vi "Teleop.vi"(10 "Match Info":T1={"Autonomous Elapsed Seconds"=0.0, "TeleOp Elapsed Seconds"=0.0, "Disabled Elapsed Seconds"=0.0, "Visited Autonomous"=FALSE, "Visited TeleOp"=FALSE, "Visited Disabled"=FALSE, "Autonomous Settings"={"Autonomous Style"=enum."Independent", "VI Refnum"=refnum}}, 11 "Call Context":T2) -> ()   [LabVIEW 2012]
doc: "This VI is called for each TeleOp packet received from the DS where the robot is not disabled. It is often used to read from the joysticks and update I/O or to update setpoints for timed control loops. It should complete and return within 20 milliseconds or it may miss DS packets."
uses:
  <vilib>/Rock Robotics/WPI/DriverStation/WPI_DriverStationDerivedRobotMode.ctl
  <vilib>/Rock Robotics/WPI/DriverStation/WPI_DriverStationMatch Info.ctl
  Robot Global Data.vi
  <vilib>/addons/control/pid/pid.llb/PID (DBL).vi
  <vilib>/Rock Robotics/WPI/Joystick/WPI_JoystickGetSetRefNum.vi
  <vilib>/addons/control/pid/NI_PID_pid.lvlib
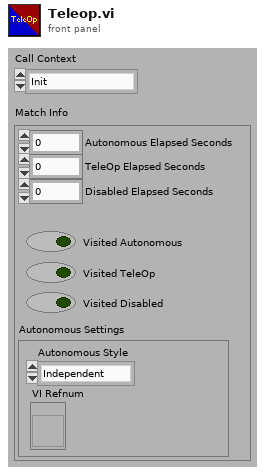
[diagram p1: front panel]
types:
  T1 = typedef "WPI_DriverStationMatch Info.ctl" = cluster{"Autonomous Elapsed Seconds":dbl, "TeleOp Elapsed Seconds":dbl, "Disabled Elapsed Seconds":dbl, "Visited Autonomous":bool, "Visited TeleOp":bool, "Visited Disabled":bool, "Autonomous Settings":cluster{"Autonomous Style":enum16{"Iterative", "Independent"}, "VI Refnum":refnum<vi>}}
  T2 = typedef "WPI_DriverStationDerivedRobotMode.ctl" = enum16{"Init", "Execute", "Stop"}
  T3 = cluster{"proportional gain (Kc)":dbl, "integral time (Ti, min)":dbl, "derivative time (Td, min)":dbl}
  T4 = typedef "WPI_JoystickDevRef.ctl" = cluster{"Device":T5}
  T5 = typedef "WPI_JoystickDeviceEnum.ctl" = enum16{"USB 1", "USB 2", "USB 3", "USB 4", "Kinect 1", "Kinect 2"}
  T6 = typedef "WPI_JoystickButtonState.ctl" = cluster{"Button 1":bool, "Button 2":bool, "Button 3":bool, "Button 4":bool, "Button 5":bool, "Button 6":bool, "Button 7":bool, "Button 8":bool, "Button 9":bool, "Button 10":bool, "Button 11":bool, "Button 12":bool}
  T7 = cluster{"axis 1 (x)":dbl, "axis 2 (y)":dbl, "axis 3 (throttle)":dbl, "axis 4":dbl, "axis 5":dbl, "axis 6":dbl}
  T8 = typedef "WPI_MotorControlDeviceRef.ctl" = cluster{"DeviceStatus":errorcluster, "Type":enum16{"PWM", "CAN"}, "PWM":cluster{"Digital Module":T9, "PWM Channel":T10, "DeadBand":T11}, "CAN":cluster{"Device Number":u8, "Control Mode":T12, "Semaphore":T13, "Max Vout":dbl}, "Invert":bool, "TransformRef":T14, "InvTransformRef":T14}
  T9 = typedef "FPGA_TypedefDigitalModule.ctl" = enum16{"Digital Module 1", "Digital Module 2"}
  T10 = typedef "FPGA_DIOPWMChannel.ctl" = enum8{"PWM 1", "PWM 2", "PWM 3", "PWM 4", "PWM 5", "PWM 6", "PWM 7", "PWM 8", "PWM 9", "PWM 10", "Invalid"}
  T11 = typedef "WPI_PWMDeadband.ctl" = cluster{"Name":string, "maxPositivePwm":i32, "minPositivePwm":i32, "centerPwm":i32, "maxNegativePwm":i32, "minNegativePwm":i32, "angularRange":u16}
  T12 = typedef "WPI_CANJaguar_ControlMode.ctl" = enum8{"Percent VBus", "Current", "Speed", "Position", "Voltage"}
  T13 = typedef "Semaphore RefNum" = refnum<k1>
  T14 = typedef "WPI_PWMTransform_ConPane.ctl" = refnum<vi>
  T15 = typedef "WPI_AnalogChannelDevRef.ctl" = cluster{"DevStatus":errorcluster, "Analog Module":T16, "Analog Channel":T17}
  T16 = typedef "FPGA_TypedefAnalogModule.ctl" = enum16{"Analog Module 1", "Analog Module 2"}
  T17 = typedef "FPGA_AIChannel.ctl" = enum8{"AI 1", "AI 2", "AI 3", "AI 4", "AI 5", "AI 6", "AI 7", "AI 8", "Invalid"}
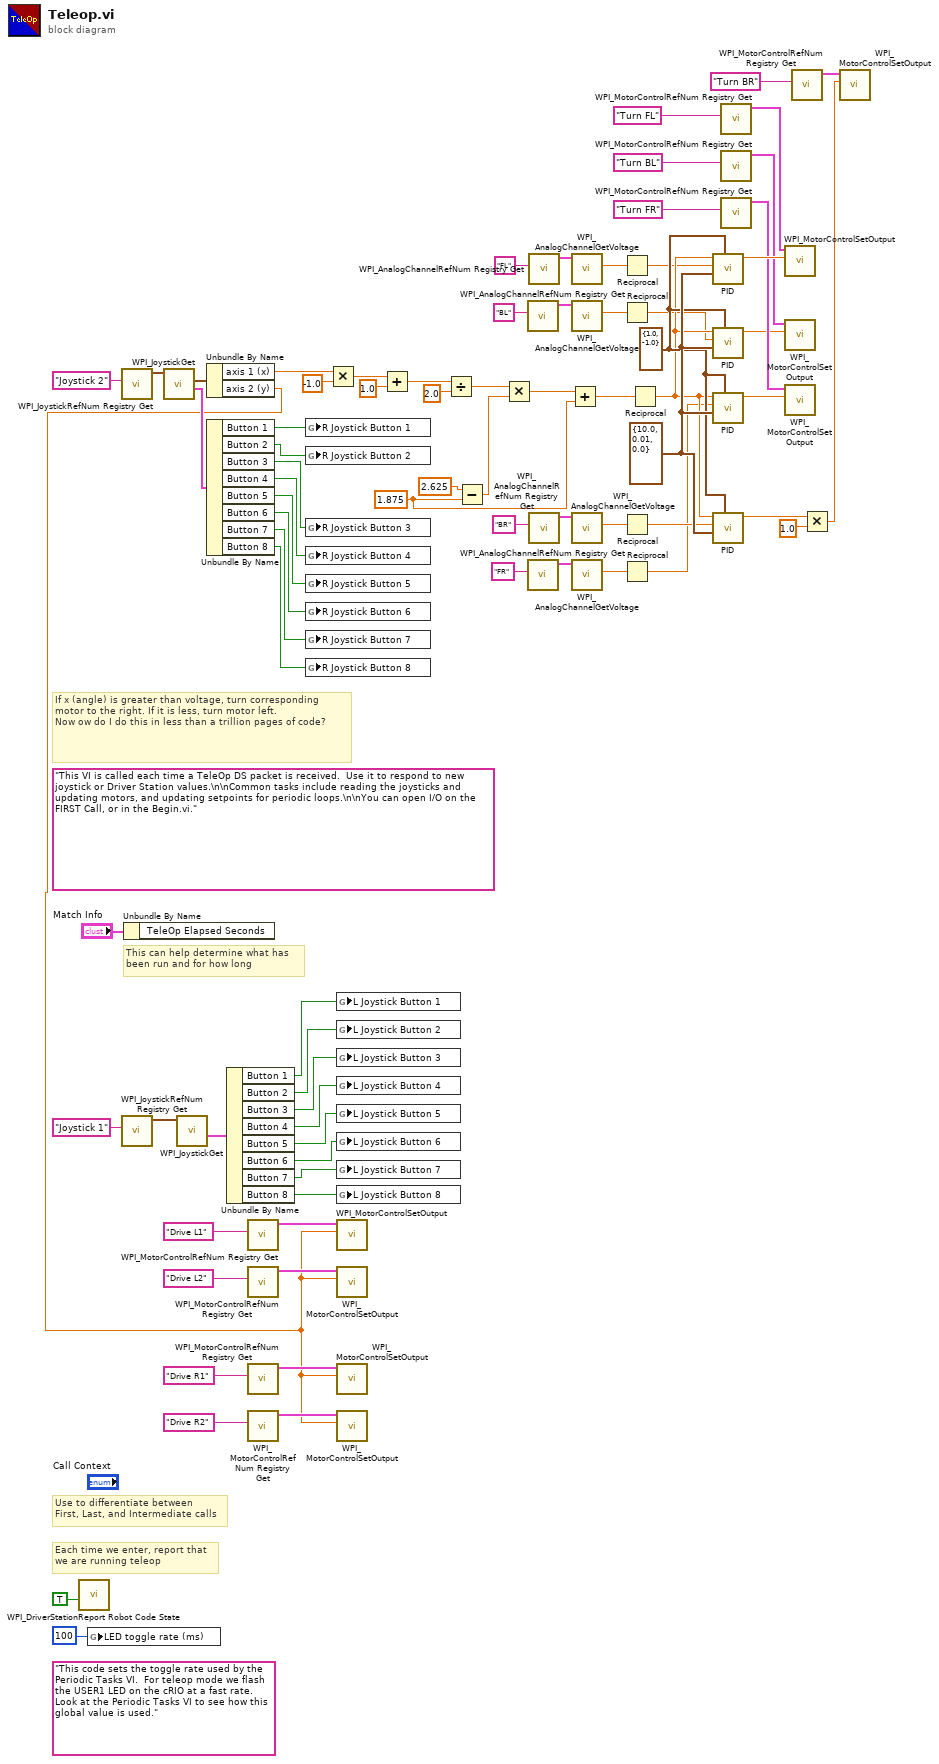
[diagram p0: block diagram]
diagram:
  w21 = T3 {"proportional gain (Kc)"=10.0, "integral time (Ti, min)"=0.01, "derivative time (Td, min)"=0.0} ("PID gains")
  w20 = cluster{"output high":dbl, "output low":dbl} {"output high"=1.0, "output low"=-1.0} ("output range")
  w19 = 1.875 ("y")
  (unwired) "This code sets the toggle rate used by the Periodic Tasks VI.  For teleop mode we flash the USER1 LED on the cRIO at a fast rate.  Look at the Periodic Tasks VI to see how this global value is used."
  (unwired) "This VI is called each time a TeleOp DS packet is received.  Use it to respond to new joystick or Driver Station values.\n\nCommon tasks include reading the joysticks and updating motors, and updating setpoints for periodic loops.\n\nYou can open I/O on the FIRST Call, or in the Begin.vi."
  # "If x (angle) is greater than voltage, turn corresponding motor to the right. If it is less, turn motor left.\nNow ow do I do this in less than a trillion pages of code?"
  # "Each time we enter, report that\nwe are running teleop"
  # "Use to differentiate between\nFirst, Last, and Intermediate calls"
  # "This can help determine what has\nbeen run and for how long"
  n1 = call <vilib>:"WPI_DriverStationReport Robot Code State.vi"("TeleOp"=TRUE ("Autonomous")) -> ()  [unwired: 10 in, 1 out]
  n2 = global write "Robot Global Data.vi" "LED toggle rate (ms)"(u32 100 ("LED ms toggle rate")) -> ()
  n3 = call <vilib>:"WPI_JoystickRefNum Registry Get.vi"("refnum name"="Joystick 2") -> ("JoystickDevRef"=w73:T4)  [unwired: 1 in, 9 out]
  n4 = call <vilib>:"WPI_JoystickRefNum Registry Get.vi"("refnum name"="Joystick 1") -> ("JoystickDevRef"=w78:T4)  [unwired: 1 in, 9 out]
  n5 = Unbundle By Name("Match Info") -> ()  [unwired: 1 out]
  n6 = call <vilib>:"WPI_JoystickGet.vi"("JoystickDevRef"=w73) -> ("Buttons"=w72:T6, "Axes"=w75:T7)  [unwired: 1 in, 4 out]
  n7 = call <vilib>:"WPI_JoystickGet.vi"("JoystickDevRef"=w78) -> ("Buttons"=w71:T6)  [unwired: 1 in, 5 out]
  n8 = Unbundle By Name(w75) -> ("axis 1 (x)"=w11:dbl, "axis 2 (y)"=w1:dbl)
  n9 = Unbundle By Name(w72) -> ("Button 1"=w62:bool, "Button 2"=w61:bool, "Button 3"=w60:bool, "Button 4"=w59:bool, "Button 5"=w58:bool, "Button 6"=w57:bool, "Button 7"=w56:bool, "Button 8"=w55:bool)
  n10 = Unbundle By Name(w71) -> ("Button 1"=w70:bool, "Button 2"=w69:bool, "Button 3"=w68:bool, "Button 4"=w67:bool, "Button 5"=w66:bool, "Button 6"=w65:bool, "Button 7"=w64:bool, "Button 8"=w63:bool)
  n11 = call <vilib>:"WPI_MotorControlRefNum Registry Get.vi"("refnum name"="Drive L1") -> ("MotorControlDevRef"=w47:T8)  [unwired: 9 in, 1 out]
  n12 = call <vilib>:"WPI_MotorControlRefNum Registry Get.vi"("refnum name"="Drive L2") -> ("MotorControlDevRef"=w46:T8)  [unwired: 9 in, 1 out]
  n13 = call <vilib>:"WPI_MotorControlRefNum Registry Get.vi"("refnum name"="Drive R1") -> ("MotorControlDevRef"=w45:T8)  [unwired: 9 in, 1 out]
  n14 = call <vilib>:"WPI_MotorControlRefNum Registry Get.vi"("refnum name"="Drive R2") -> ("MotorControlDevRef"=w44:T8)  [unwired: 9 in, 1 out]
  n15 = global write "Robot Global Data.vi" "R Joystick Button 1"(w62) -> ()
  n16 = global write "Robot Global Data.vi" "R Joystick Button 2"(w61) -> ()
  n17 = global write "Robot Global Data.vi" "R Joystick Button 3"(w60) -> ()
  n18 = global write "Robot Global Data.vi" "R Joystick Button 4"(w59) -> ()
  n19 = global write "Robot Global Data.vi" "R Joystick Button 5"(w58) -> ()
  n20 = global write "Robot Global Data.vi" "R Joystick Button 6"(w57) -> ()
  n21 = global write "Robot Global Data.vi" "R Joystick Button 7"(w56) -> ()
  n22 = global write "Robot Global Data.vi" "R Joystick Button 8"(w55) -> ()
  n23 = Multiply(x=w11, y=-1.0) -> (x*y=w10:dbl)
  n24 = global write "Robot Global Data.vi" "L Joystick Button 1"(w70) -> ()
  n25 = global write "Robot Global Data.vi" "L Joystick Button 2"(w69) -> ()
  n26 = global write "Robot Global Data.vi" "L Joystick Button 3"(w68) -> ()
  n27 = global write "Robot Global Data.vi" "L Joystick Button 4"(w67) -> ()
  n28 = global write "Robot Global Data.vi" "L Joystick Button 5"(w66) -> ()
  n29 = global write "Robot Global Data.vi" "L Joystick Button 6"(w65) -> ()
  n30 = global write "Robot Global Data.vi" "L Joystick Button 7"(w64) -> ()
  n31 = global write "Robot Global Data.vi" "L Joystick Button 8"(w63) -> ()
  n32 = call <vilib>:"WPI_MotorControlSetOutput.vi"("Output"=w1, "MotorControlDevRef"=w47) -> ()  [unwired: 7 in, 3 out]
  n33 = call <vilib>:"WPI_MotorControlSetOutput.vi"("Output"=w1, "MotorControlDevRef"=w46) -> ()  [unwired: 7 in, 3 out]
  n34 = call <vilib>:"WPI_MotorControlSetOutput.vi"("Output"=w1, "MotorControlDevRef"=w45) -> ()  [unwired: 7 in, 3 out]
  n35 = call <vilib>:"WPI_MotorControlSetOutput.vi"("Output"=w1, "MotorControlDevRef"=w44) -> ()  [unwired: 7 in, 3 out]
  n36 = Add(x=w10, y=1.0) -> (x+y=w42:dbl)
  n37 = Divide(x=w42, y=2.0) -> (x/y=w38:dbl)
  n38 = Subtract(x=2.625, y=w19) -> (x-y=w39:dbl)
  n39 = Multiply(x=w38, y=w39) -> (x*y=w40:dbl)
  n40 = call <vilib>:"WPI_AnalogChannelRefNum Registry Get.vi"("refnum name"="BL") -> ("AIDeviceRef"=w26:T15)  [unwired: 9 in, 1 out]
  n41 = call <vilib>:"WPI_AnalogChannelRefNum Registry Get.vi"("refnum name"="FR") -> ("AIDeviceRef"=w31:T15)  [unwired: 9 in, 1 out]
  n42 = call <vilib>:"WPI_AnalogChannelRefNum Registry Get.vi"("refnum name"="FL") -> ("AIDeviceRef"=w36:T15)  [unwired: 9 in, 1 out]
  n43 = call <vilib>:"WPI_AnalogChannelRefNum Registry Get.vi"("refnum name"="BR") -> ("AIDeviceRef"=w54:T15)  [unwired: 9 in, 1 out]
  n44 = Add(x=w40, y=w19) -> (x+y=w9:dbl)
  n45 = call <vilib>:"WPI_AnalogChannelGetVoltage.vi"("AIDeviceRef"=w36) -> ("Voltage"=w3:dbl)  [unwired: 8 in, 2 out]
  n46 = call <vilib>:"WPI_AnalogChannelGetVoltage.vi"("AIDeviceRef"=w26) -> ("Voltage"=w7:dbl)  [unwired: 8 in, 2 out]
  n47 = call <vilib>:"WPI_AnalogChannelGetVoltage.vi"("AIDeviceRef"=w54) -> ("Voltage"=w14:dbl)  [unwired: 8 in, 2 out]
  n48 = call <vilib>:"WPI_AnalogChannelGetVoltage.vi"("AIDeviceRef"=w31) -> ("Voltage"=w5:dbl)  [unwired: 8 in, 2 out]
  n49 = Reciprocal(x=w3) -> (1/x=w2:dbl)
  n50 = Reciprocal(x=w7) -> (1/x=w6:dbl)
  n51 = Reciprocal(x=w14) -> (1/x=w13:dbl)
  n52 = Reciprocal(x=w5) -> (1/x=w4:dbl)
  n53 = Reciprocal(x=w9) -> (1/x=w8:dbl)
  n54 = call-poly <vilib>:"PID.vi"("output range"=w20, "PID gains"=w21, "process variable"=w2, "setpoint"=w8) -> ("output"=w33:dbl)  [unwired: 6 in, 1 out]
  n55 = call-poly <vilib>:"PID.vi"("output range"=w20, "PID gains"=w21, "process variable"=w6, "setpoint"=w8) -> ("output"=w23:dbl)  [unwired: 6 in, 1 out]
  n56 = call-poly <vilib>:"PID.vi"("output range"=w20, "PID gains"=w21, "process variable"=w4, "setpoint"=w8) -> ("output"=w28:dbl)  [unwired: 6 in, 1 out]
  n57 = call-poly <vilib>:"PID.vi"("output range"=w20, "PID gains"=w21, "process variable"=w13, "setpoint"=w8) -> ("output"=w16:dbl)  [unwired: 6 in, 1 out]
  n58 = call <vilib>:"WPI_MotorControlRefNum Registry Get.vi"("refnum name"="Turn FL") -> ("MotorControlDevRef"=w32:T8)  [unwired: 9 in, 1 out]
  n59 = call <vilib>:"WPI_MotorControlRefNum Registry Get.vi"("refnum name"="Turn BL") -> ("MotorControlDevRef"=w22:T8)  [unwired: 9 in, 1 out]
  n60 = call <vilib>:"WPI_MotorControlRefNum Registry Get.vi"("refnum name"="Turn FR") -> ("MotorControlDevRef"=w27:T8)  [unwired: 9 in, 1 out]
  n61 = call <vilib>:"WPI_MotorControlSetOutput.vi"("Output"=w33, "MotorControlDevRef"=w32) -> ()  [unwired: 7 in, 3 out]
  n62 = call <vilib>:"WPI_MotorControlSetOutput.vi"("Output"=w23, "MotorControlDevRef"=w22) -> ()  [unwired: 7 in, 3 out]
  n63 = call <vilib>:"WPI_MotorControlSetOutput.vi"("Output"=w28, "MotorControlDevRef"=w27) -> ()  [unwired: 7 in, 3 out]
  n64 = call <vilib>:"WPI_MotorControlRefNum Registry Get.vi"("refnum name"="Turn BR") -> ("MotorControlDevRef"=w37:T8)  [unwired: 9 in, 1 out]
  n65 = Multiply(x=w16, y=1.0) -> (x*y=w15:dbl)
  n66 = call <vilib>:"WPI_MotorControlSetOutput.vi"("Output"=w15, "MotorControlDevRef"=w37) -> ()  [unwired: 7 in, 3 out]
